vi "MeasurementServer_Stream_Error.vi"(8 "error in (no error)":errorcluster, 10 "ErrorOutData":T1, 11 "gRPCid":T2) -> (0 "error out":errorcluster, 3 "gRPCid out":T2)   [LabVIEW 2019, in "labview-grpc-measurement-server.lvlib"]
uses:
  labview-grpc-measurement-server.lvlib
  MeasurementServer_gRPCid.ctl
  MeasurementServer_ErrorOutData.ctl
  <vilib>/Utility/error.llb/Error Cluster From Error Code.vi
  <vilib>/ErrorRing/Error Ring.xnode
  home/lvuser/liblabview_measurement_server.so
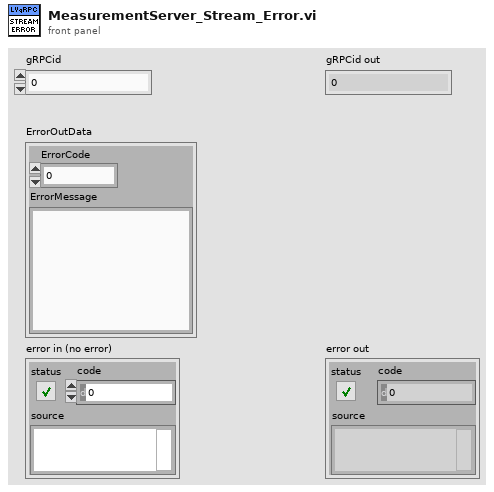
[diagram p1: front panel]
types:
  T1 = typedef "labview-grpc-measurement-server.lvlib/MeasurementServer_ErrorOutData.ctl" = cluster{"ErrorCode":i32, "ErrorMessage":string}
  T2 = typedef "labview-grpc-measurement-server.lvlib/MeasurementServer_gRPCid.ctl" = u64
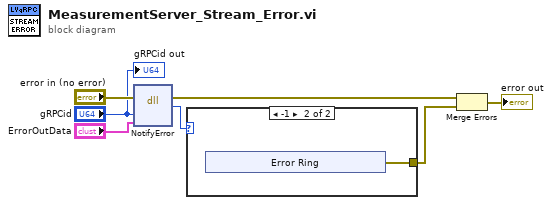
[diagram p0: block diagram]
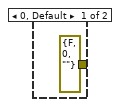
[diagram p2: hidden frame]
diagram:
  n1 = dll-call lib="home/lvuser/liblabview_measurement_server.so" fn="NotifyError"(error in="error in (no error)", "id"="gRPCid", "data"="ErrorOutData") -> (error out=w3:errorcluster, "return type"=w2:i32)  [unwired: 4 in, 1 out]
  n2 = case shown="-1" w2 {
    tunnel: [errorcluster {"status"=FALSE, "code"=0, "source"=""} ("error constant") w9] -> w4
    frame 0, Default {
    }
    frame -1 {
      n3 = xnode "Error Ring"() -> ("error out"=w9:errorcluster)
    }
  }
  n4 = Merge Errors(w3, w4) -> (→"error out":errorcluster)
  "gRPCid out" <- "gRPCid"
